vi "Override Error.vi"(10 "Error":errorcluster, 11 "TEMPLATE Event in":refnum<class "TEMPLATE Event.lvclass">) -> (3 "TEMPLATE Event out":refnum<class "TEMPLATE Event.lvclass">)   [LabVIEW 2021, in "_Template.lvlib" / "Templates.lvlib" / "TEMPLATE Event.lvlib" / "TEMPLATE Event.lvclass"]
uses:
  TEMPLATE Event.lvclass
  TEMPLATE Event.lvclass/TEMPLATE Event.ctl
  <vilib>/Nathan Davis/jettl/jettl/Event/Event.lvclass
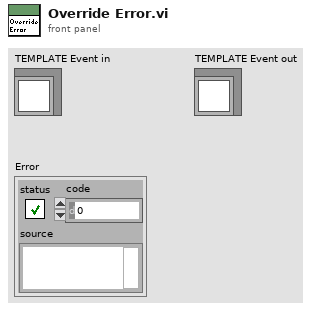
[diagram p1: front panel]
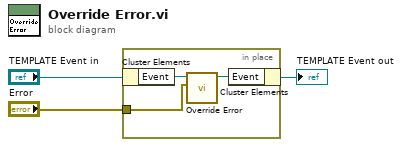
[diagram p0: block diagram]
diagram:
  n1 = in-place {
    in-place-border: "Error" -> [w4]
    n2 = in-place-cluster #1("TEMPLATE Event in") -> ("Event"=w6:refnum<class "Event.lvclass">)
    n3 = call-dynamic "Override Error.vi"("Error"=w4, "jettl Msg Override Error in"=w6) -> ("jettl Msg Override Error out"=w5:refnum<class "Event.lvclass">)  [unwired: 9 in]
    n4 = in-place-cluster #1("Event"=w5) -> (→"TEMPLATE Event out":refnum<class "TEMPLATE Event.lvclass">)
  }
